vi "subVI_Strain_Ass.vi"(2 "속도":dbl=50000.0, 3 "샘플 개수":i32=1000, 4 "timeout (s)":dbl=10.0 caption="타임아웃(초)" format="%0.2f", 5 "error in":errorcluster caption="에러 입력", 7 "stop (T)":bool=TRUE caption="정지(T)") -> (14 "task out":refnum<k21> caption="태스크 출력", 15 "data":dynamicdata(graph) caption="데이터", 19 "error out":errorcluster caption="에러 출력")   [LabVIEW 2013]
doc: "NI-DAQmx를 사용하여 태스크를 생성, 편집, 실행합니다. NI-DAQmx가 지원하는 디바이스의 완전한 리스트는 NI-DAQ Readme를 참조하십시오.\n\n이 익스프레스 VI를 블록다이어그램에 놓으면 DAQ 어시스턴트가 시작되어 새로운 태스크를 생성합니다, 태스크를 생성한 후, DAQ 어시스턴트 익스프레스 VI를 더블 클릭하여 해당 태스크를 편집할 수 있습니다. 연속적인 측정 또는 생성을 위해서는 DAQ 어시스턴트 익스프레스 주위에 while 루프를 놓습니다.\n\n연속적인 단일 포인트 입력 또는 출력의 경우 DAQ 어시스턴트 익스프레스 VI는 최적의 성능을 제공하지 않을 수도 있습니다. 높은 성능을 가진 단일 포인트 I/O 어플리케이션을 생성하는 기술에 대한 예제는 examples\\DAQmx\\Analog In\\Measure Voltage.llb의 Cont Acq&Graph Voltage-Single Point Optimization VI를 참조하십시오."
uses:
  <vilib>/DAQmx/read.llb/DAQmx Read.vi
  <vilib>/DAQmx/read.llb/DAQmx Read (Analog 1D Wfm NChan NSamp).vi
  <vilib>/DAQmx/create/channels.llb/DAQmx Create Channel (TEDS-AI-Strain-Strain Gage).vi
  <vilib>/DAQmx/create/channels.llb/DAQmx Create Channel (AI-Strain-Strain Gage).vi
  <vilib>/DAQmx/configure/timing.llb/DAQmx Timing (Sample Clock).vi
  <vilib>/DAQmx/configure/trigger.llb/DAQmx Trigger.vi
  <vilib>/DAQmx/configure/trigger.llb/DAQmx Start Trigger (Digital Edge).vi
  <vilib>/DAQmx/miscellaneous.llb/DAQmx Fill In Error Info.vi
  <resource>/objmgr/daqmx.rc
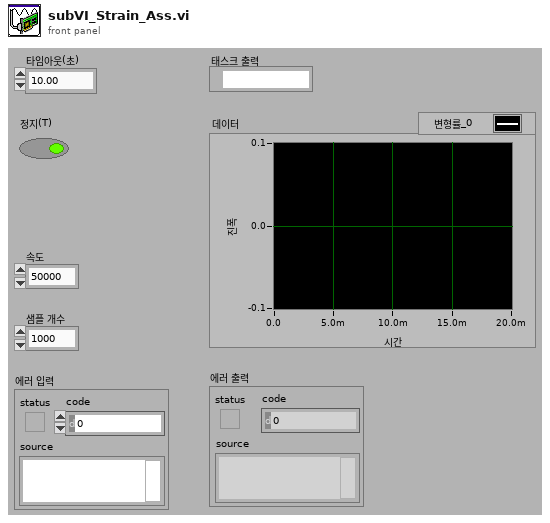
[diagram p1: front panel]
types:
  T1 = cluster{"lead resistance":dbl, "initial bridge voltage":dbl, "excitation source":i32, "excitation value":dbl}
  T2 = cluster{"strain configuration":i32, "lead resistance":dbl, "initial bridge voltage":dbl, "excitation source":i32, "excitation value":dbl}
  T3 = cluster{"gage factor":dbl, "nominal gage resistance":dbl, "poisson ratio":dbl}
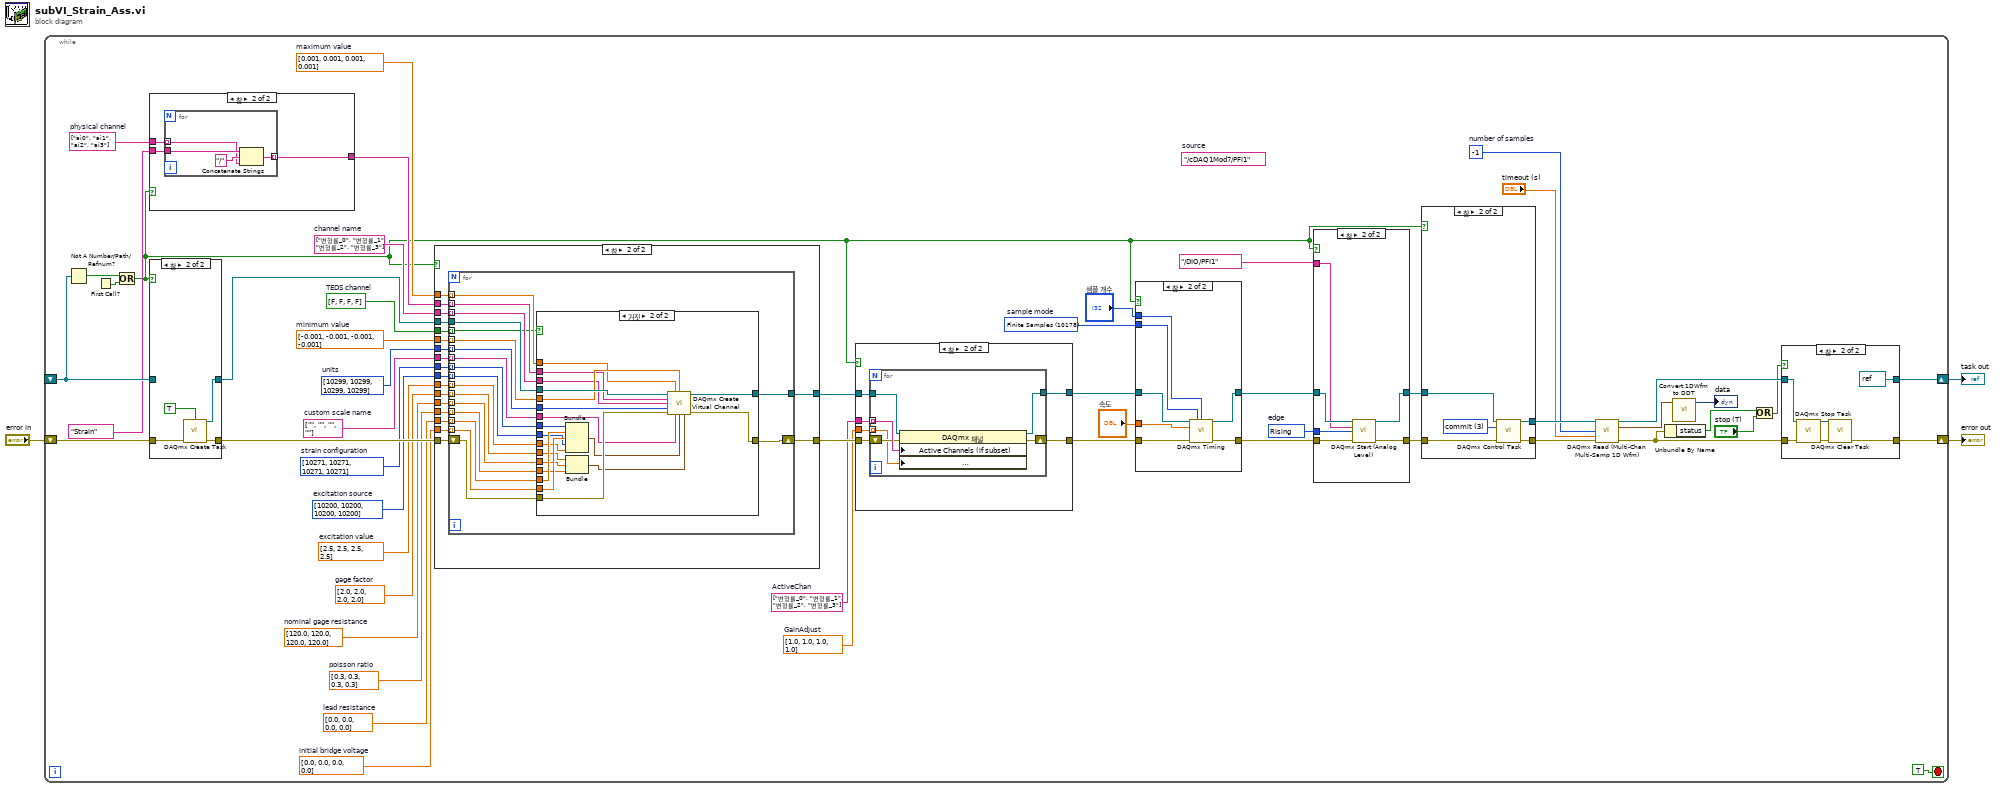
[diagram p0: block diagram]
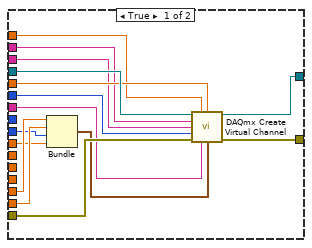
[diagram p8: hidden frame]
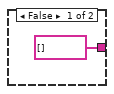
[diagram p9: hidden frame]
diagram:
  n1 = while {
    shift-right: [w11] -> w1
    shift-left: _ -> [w53]
    shift-right: [w9] -> w2
    shift-left: "error in" -> [w54]
    stop <- TRUE stop-if-true
    w15 = -1  # number of samples
    w21 = 10280 items=["Rising"=10280, "Falling"=10171]  # edge
    (unwired) "/cDAQ1Mod7/PFI1"  # source
    w24 = 10178 items=["Finite Samples"=10178, "Continuous Samples"=10123, "Hardware Timed Single Point"=12522]  # sample mode
    w29 = dbl[] [1.0, 1.0, 1.0, 1.0]  # GainAdjust
    w30 = string[] ["변형률_0", "변형률_1", "변형률_2", "변형률_3"]  # ActiveChan
    w33 = bool[] [FALSE, FALSE, FALSE, FALSE]  # TEDS channel
    w34 = dbl[] [0.3, 0.3, 0.3, 0.3]  # poisson ratio
    w35 = dbl[] [120.0, 120.0, 120.0, 120.0]  # nominal gage resistance
    w36 = dbl[] [2.0, 2.0, 2.0, 2.0]  # gage factor
    w37 = dbl[] [2.5, 2.5, 2.5, 2.5]  # excitation value
    w38 = i32[] [10200, 10200, 10200, 10200] items=["Internal"=10200, "External"=10167, "None"=10230]  # excitation source
    w39 = dbl[] [0.0, 0.0, 0.0, 0.0]  # initial bridge voltage
    w41 = i32[] [10271, 10271, 10271, 10271] items=["Full Bridge I"=10183, "Full Bridge II"=10184, "Full Bridge III"=10185, "Half Bridge I"=10188, "Half Bridge II"=10189, "Quarter Bridge I"=10271, "Quarter Bridge II"=10272]  # strain configuration
    w40 = dbl[] [0.0, 0.0, 0.0, 0.0]  # lead resistance
    w42 = string[] ["", "", "", ""]  # custom scale name
    w43 = i32[] [10299, 10299, 10299, 10299] items=["Strain"=10299, "From Custom Scale"=10065]  # units
    w44 = string[] ["변형률_0", "변형률_1", "변형률_2", "변형률_3"]  # channel name
    w46 = dbl[] [0.001, 0.001, 0.001, 0.001]  # maximum value
    w47 = dbl[] [-0.001, -0.001, -0.001, -0.001]  # minimum value
    w50 = string[] ["ai0", "ai1", "ai2", "ai3"]  # physical channel
    n2 = Not A Number/Path/Refnum?(number/path/refnum=w53) -> (NaN/Path/Refnum?=w52:bool)
    n3 = First Call?() -> (First Call?: T/F=w55:bool)
    n4 = Or(x=w52, y=w55) -> (x .or. y?=w20:bool)
    n5 = case "케이스 구조" shown="참" w20 {
      tunnel: [string[] [] w181] -> w45
      tunnel: tag "Strain" ("디바이스 이름") -> [_ w180]
      tunnel: w50 -> [_ w179]
      frame False {
      }
      frame True {
        n6 = for "For 루프" {
          tunnel: [w185] -> w181 mode=indexing
          tunnel: w180 -> [w184]
          tunnel: w179 -> [w182] mode=indexing
          n7 = Concatenate Strings(w184, "/" ("string"), w182) -> (w185:string)
        }
      }
    }
    n8 = case "케이스 구조" shown="참" w20 {
      tunnel: [w187 w191] -> w49
      tunnel: w53 -> [w187 _]
      tunnel: [w186 w190] -> w48
      tunnel: w54 -> [w186 w188]
      frame False {
      }
      frame True {
        n9 = call <vilib>:"DAQmx Create Task.vi"("auto cleanup"=TRUE, "error in"=w188) -> ("task out"=w191:refnum<k21>, "error out"=w190:errorcluster)  [unwired: 12 in]
      }
    }
    n10 = case "케이스 구조" shown="참" w20 {
      tunnel: [w104 w121] -> w32
      tunnel: w49 -> [w104 w123]
      tunnel: [w103 w120] -> w31
      tunnel: w48 -> [w103 w122]
      tunnel: w47 -> [_ w119]
      tunnel: w46 -> [_ w118]
      tunnel: w45 -> [_ w117]
      tunnel: w44 -> [_ w116]
      tunnel: w43 -> [_ w115]
      tunnel: w42 -> [_ w114]
      tunnel: w41 -> [_ w113]
      tunnel: w40 -> [_ w112]
      tunnel: w39 -> [_ w111]
      tunnel: w38 -> [_ w110]
      tunnel: w37 -> [_ w109]
      tunnel: w36 -> [_ w108]
      tunnel: w35 -> [_ w107]
      tunnel: w34 -> [_ w106]
      tunnel: w33 -> [_ w105]
      frame False {
      }
      frame True {
        n11 = for "For 루프" {
          tunnel: w123 -> [w142]
          tunnel: [w140] -> w121
          tunnel: w119 -> [w138] mode=indexing
          tunnel: w118 -> [w137] mode=indexing
          tunnel: w117 -> [w136] mode=indexing
          tunnel: w116 -> [w135] mode=indexing
          shift-right: [w139] -> w120
          shift-left: w122 -> [w141]
          tunnel: w115 -> [w134] mode=indexing
          tunnel: w114 -> [w133] mode=indexing
          tunnel: w113 -> [w132] mode=indexing
          tunnel: w112 -> [w131] mode=indexing
          tunnel: w111 -> [w130] mode=indexing
          tunnel: w110 -> [w129] mode=indexing
          tunnel: w109 -> [w128] mode=indexing
          tunnel: w108 -> [w127] mode=indexing
          tunnel: w107 -> [w126] mode=indexing
          tunnel: w106 -> [w125] mode=indexing
          tunnel: w105 -> [w124] mode=indexing
          n12 = case "케이스 구조" shown="거짓" w124 {
            tunnel: w142 -> [w157 w177]
            tunnel: w141 -> [w156 w176]
            tunnel: [w155 w175] -> w140
            tunnel: [w154 w174] -> w139
            tunnel: w138 -> [w153 w173]
            tunnel: w137 -> [w152 w172]
            tunnel: w136 -> [w151 w171]
            tunnel: w135 -> [w150 w170]
            tunnel: w134 -> [w148 w168]
            tunnel: w133 -> [w147 w167]
            tunnel: w132 -> [_ w166]
            tunnel: w131 -> [w146 w165]
            tunnel: w130 -> [w145 w164]
            tunnel: w129 -> [w144 w163]
            tunnel: w128 -> [w143 w162]
            tunnel: w127 -> [_ w161]
            tunnel: w126 -> [_ w160]
            tunnel: w125 -> [_ w159]
            frame True {
              n13 = Bundle("lead resistance"=w146, "initial bridge voltage"=w145, "excitation source"=w144, "excitation value"=w143) -> (w149:T1)  [unwired: 1 in]
              n14 = call-poly <vilib>:"DAQmx Create Virtual Channel.vi"("task in"=w157, "maximum value"=w152, "minimum value"=w153, "physical channels"=w151, "name to assign"=w150, "units"=w148, "error in"=w156, "custom scale name"=w147, "bridge information"=w149) -> ("task out"=w155:refnum<k21>, "error out"=w154:errorcluster)  [unwired: 5 in]
            }
            frame False {
              n15 = Bundle("strain configuration"=w166, "lead resistance"=w165, "initial bridge voltage"=w164, "excitation source"=w163, "excitation value"=w162) -> (w169:T2)  [unwired: 1 in]
              n16 = Bundle("gage factor"=w161, "nominal gage resistance"=w160, "poisson ratio"=w159) -> (w158:T3)  [unwired: 1 in]
              n17 = call-poly <vilib>:"DAQmx Create Virtual Channel.vi"("task in"=w177, "maximum value"=w172, "minimum value"=w173, "physical channels"=w171, "name to assign"=w170, "units"=w168, "error in"=w176, "custom scale name"=w167, "bridge information"=w169, "strain gage information"=w158) -> ("task out"=w175:refnum<k21>, "error out"=w174:errorcluster)  [unwired: 4 in]
            }
          }
        }
      }
    }
    n18 = case "케이스 구조" shown="참" w20 {
      tunnel: [w90 w93] -> w28
      tunnel: w32 -> [w90 w96]
      tunnel: [w89 w94] -> w27
      tunnel: w31 -> [w89 w95]
      tunnel: w30 -> [_ w92]
      tunnel: w29 -> [_ w91]
      frame False {
      }
      frame True {
        n19 = for "For 루프" {
          tunnel: w96 -> [w102]
          shift-right: [w100] -> w94
          shift-left: w95 -> [w98]
          tunnel: [w101] -> w93
          tunnel: w92 -> [w99] mode=indexing
          tunnel: w91 -> [w97] mode=indexing
          n20 = property class="DAQmx 채널"(reference=w102, error in=w98, "Active Channels (if subset)"=w99, "Analog Input:General Properties:Signal Conditioning:Bridge:Shunt Cal:Gain Adjustment"=w97) -> (reference out=w101:refnum<k21>, error out=w100:errorcluster)
        }
      }
    }
    n21 = case "케이스 구조" shown="참" w20 {
      tunnel: [w81 w83] -> w23
      tunnel: w28 -> [w81 w86]
      tunnel: [w80 w82] -> w22
      tunnel: w27 -> [w80 w84]
      tunnel: "샘플 개수" -> [_ w88]
      tunnel: w24 -> [_ w87]
      tunnel: "속도" -> [_ w85]
      frame False {
      }
      frame True {
        n22 = call-poly <vilib>:"DAQmx Timing.vi"("task/channels in"=w86, "sample mode"=w87, "samples per channel"=w88, "rate"=w85, "error in"=w84) -> ("task out"=w83:refnum<k21>, "error out"=w82:errorcluster)  [unwired: 9 in]
      }
    }
    n23 = case "케이스 구조" shown="참" w20 {
      tunnel: [w73 w77] -> w19
      tunnel: w23 -> [w73 w79]
      tunnel: [w72 w76] -> w18
      tunnel: w22 -> [w72 w78]
      tunnel: tag "/DIO/PFI1" ("source") -> [_ w75]
      tunnel: w21 -> [_ w74]
      frame False {
      }
      frame True {
        n24 = call-poly "DAQmx Start (Analog Level).vi"("task/channels in"=w79, "source"=w75, "edge"=w74, "error in"=w78) -> ("task out"=w77:refnum<k21>, "error out"=w76:errorcluster)  [unwired: 10 in]
      }
    }
    n25 = case "케이스 구조" shown="참" w20 {
      tunnel: [w66 w70] -> w17
      tunnel: w19 -> [w66 w71]
      tunnel: [w65 w68] -> w16
      tunnel: w18 -> [w65 w69]
      frame False {
      }
      frame True {
        w67 = 3 items=["verify"=2, "reserve"=4, "commit"=3, "unreserve"=5, "abort"=6] ("action")
        n26 = call <vilib>:"DAQmx Control Task.vi"("task/channels in"=w71, "action"=w67, "error in"=w69) -> ("task out"=w70:refnum<k21>, "error out"=w68:errorcluster)  [unwired: 11 in]
      }
    }
    n27 = call-poly "DAQmx Read (Multi-Chan Multi-Samp 1D Wfm).vi"("task/channels in"=w17, "number of samples per channel"=w15, "timeout"="timeout (s)", "error in"=w16) -> ("task out"=w10:refnum<k21>, "data"=w14:waveform(dbl)[], "error out"=w8:errorcluster)  [unwired: 9 in]
    n28 = Unbundle By Name(w8) -> ("status"=w7:bool)
    n29 = call <vilib>:"Convert 1DWfm to DDT.vi"("Array of Waveforms"=w14) -> ("Dynamic Data Type"=→"data":dynamicdata)  [unwired: 3 in]
    n30 = Or(x=w7, y="stop (T)") -> (x .or. y?=w5:bool)
    n31 = case "케이스 구조" shown="참" w5 {
      tunnel: [w58 refnum<k21> refnum ("task in")] -> w11
      tunnel: w10 -> [w58 w64]
      tunnel: [w57 w61] -> w9
      tunnel: w8 -> [w57 w63]
      frame False {
      }
      frame True {
        n32 = call <vilib>:"DAQmx Stop Task.vi"("task/channels in"=w64, "error in"=w63) -> ("task out"=w60:refnum<k21>, "error out"=w62:errorcluster)  [unwired: 12 in]
        n33 = call <vilib>:"DAQmx Clear Task.vi"("task in"=w60, "error in"=w62) -> ("error out"=w61:errorcluster)  [unwired: 13 in]
      }
    }
  }
  "error out" <- w2
  "task out" <- w1
